vi "coin_flip.vi"() -> (2 "x >= y?":bool)   [LabVIEW 2013]
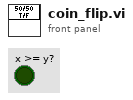
[diagram p1: front panel]
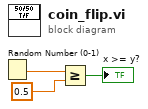
[diagram p0: block diagram]
diagram:
  n1 = Random Number (0-1)() -> (number: 0 to 1=w3:dbl)
  n2 = Greater Or Equal?(x=w3, y=0.5) -> (x >= y?=→"x >= y?":bool)
